vi "terminal.vi"() -> ()   [LabVIEW 2020]
panel:
  out "Terminal":string
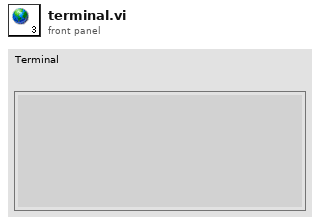
[diagram p1: front panel]
diagram:
